vi "test-popup.vi"() -> ()   [LabVIEW 2020]
uses:
  <vilib>/event_ctls.llb/eventsource.ctl
panel:
  out "Source":T1 items=["LabVIEW UI"=0, "ActiveX"=1, "User Event"=25]
  out "Time":u32
  out "VI Name":string
  out "Array":cluster{"nane":string, "data":variant}[](array[cluster])
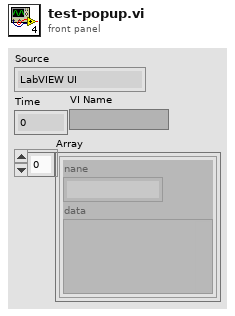
[diagram p1: front panel]
types:
  T1 = typedef "eventsource.ctl" = u32
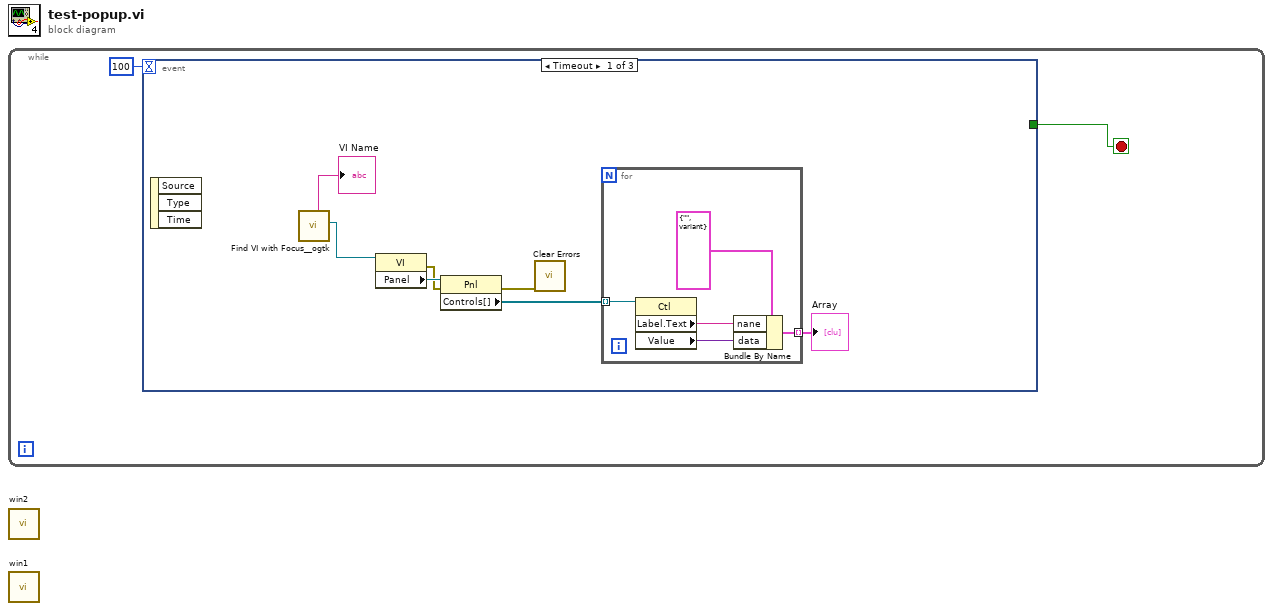
[diagram p0: block diagram]
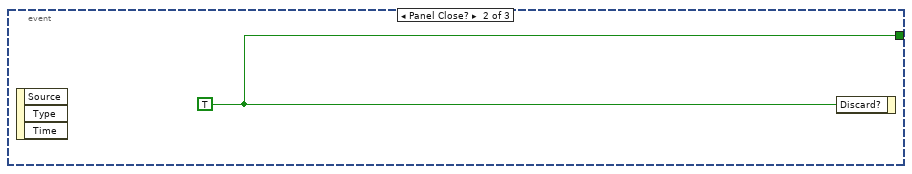
[diagram p2: hidden frame]
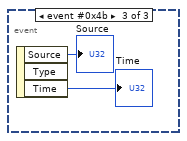
[diagram p3: hidden frame]
diagram:
  n1 = while {
    stop <- w2 stop-if-true
    n2 = event shown="[0] Timeout" {
      selector: _ -> [_ _ _]
      dyn-events: _ -> [_ _ _]
      timeout: 100 -> [_ _ _]
      tunnel: [_ w15 _] -> w2
      event Timeout {
        n3 = event-data() -> ()  [unwired: 1 in, 3 out]
        n4 = call <userlib>:"Find VI with Focus__ogtk.vi"() -> ("VI with Focus"=w8:refnum<vi>, "VI Name"=→"VI Name":string)  [unwired: 7 in, 3 out]
        n5 = property class="VI"(reference=w8) -> (error out=w4:errorcluster, "Panel"=w7:refnum<vi>)  [unwired: 1 in, 1 out]
        n6 = property class="Pnl"(reference=w7, error in=w4) -> (error out=w3:errorcluster, "Controls[]"=w6:refnum<vi>[])  [unwired: 1 out]
        n7 = call <vilib>:"Clear Errors.vi"("error in (no error)"=w3) -> ()  [unwired: 5 in, 2 out]
        n8 = for {
          tunnel: w6 -> [w14] mode=indexing
          tunnel: [w10] -> w5 mode=indexing
          n9 = property class="Ctl"(reference=w14) -> ("Label.Text"=w12:string, "Value"=w11:variant)  [unwired: 1 in, 2 out]
          n10 = Bundle By Name(cluster=cluster{"nane":string, "data":variant} {"nane"="", "data"=variant}, "nane"=w12, "data"=w11) -> (w10:cluster{"nane":string, "data":variant})
        }
        "Array" <- w5
      }
      event Panel Close? {
        w15 = TRUE ("Discard?")
        n11 = event-data() -> ()  [unwired: 1 in, 3 out]
        n12 = event-data("Discard?"=w15) -> ()  [unwired: 1 in, 1 out]
      }
      event event #0x4b {
        n13 = event-data() -> ("Source"=→"Source":T1, "Time"=→"Time":u32)  [unwired: 1 in, 1 out]
      }
    }
  }
  n14 = call "win2.vi"() -> ()  [unwired: 12 in]
  n15 = call "win1.vi"() -> ()  [unwired: 12 in]
